vi "Inspect Call.vi"(10 "Msg DVR":refnum<data-value>, 11 "TEMPLATE Actor in":refnum<class "{{Name}}Actor.lvclass">) -> (3 "TEMPLATE Actor out":refnum<class "{{Name}}Actor.lvclass">)   [LabVIEW 2020, in "_Template.lvlib" / "Templates.lvlib" / "{{Name}}Actor.lvlib" / "{{Name}}Actor.lvclass"]
uses:
  {{Name}}Actor.lvclass
  {{Name}}Actor.lvclass/{{Name}}Actor.ctl
  jettl/jettl/Message/Message.lvclass
  jettl/jettl/Actor/Actor.lvclass
  jettl/jettl/Message.ctl
  jettl/jettl/jettl.lvlib
panel:
  # "This front panel should not be manipulated."
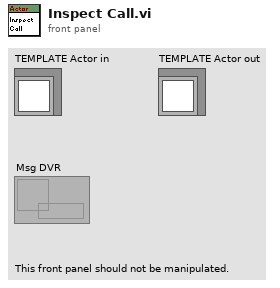
[diagram p1: front panel]
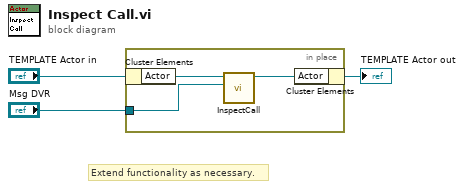
[diagram p0: block diagram]
diagram:
  # "Extend functionality as necessary."
  n1 = in-place {
    in-place-border: "Msg DVR" -> [w4]
    n2 = in-place-cluster #1("TEMPLATE Actor in") -> ("Actor"=w6:refnum<class "Actor.lvclass">)
    n3 = call-dynamic "InspectCall.vi"(10:w4, "MessageDVR in"=w6) -> ("MessageDVR out"=w5:refnum<data-value>)  [unwired: 8 in, 1 out]
    n4 = in-place-cluster #1("Actor"=w5) -> (→"TEMPLATE Actor out":refnum<class "{{Name}}Actor.lvclass">)
  }
